vi "myRIO_BRig_RT_dataTrial_activeRecording.vi"() -> (2 "output_activeRecording":i32)   [LabVIEW 2014]
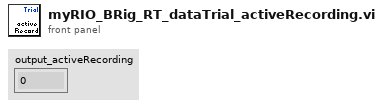
[diagram p1: front panel]
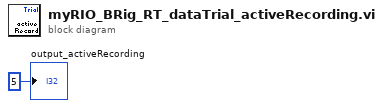
[diagram p0: block diagram]
diagram:
  "output_activeRecording" <- 5 ("output_iBlock")
